vi "test - click2.vi"() -> ()   [LabVIEW 2020]
uses:
  <vilib>/Utility/miscctls.llb/LVPositionTypeDef.ctl
  ui-testing.lvlib
  User32.dll
panel:
  out "Position":T1
  in  "OK Button":bool
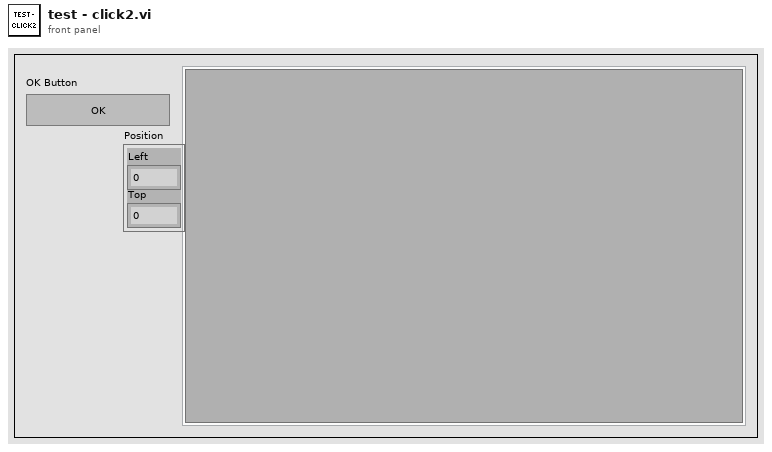
[diagram p1: front panel]
types:
  T1 = typedef "LVPositionTypeDef.ctl" = cluster{"Left":i32, "Top":i32}
  T2 = typedef "LVPointTypeDef.ctl" = cluster{"Horizontal":i16, "Vertical":i16}
  T3 = typedef "LVRectTypeDef.ctl" = cluster{"left":i16, "top":i16, "right":i16, "bottom":i16}
  T4 = typedef "LVBoundsTypeDef.ctl" = cluster{"Width":u32, "Height":u32}
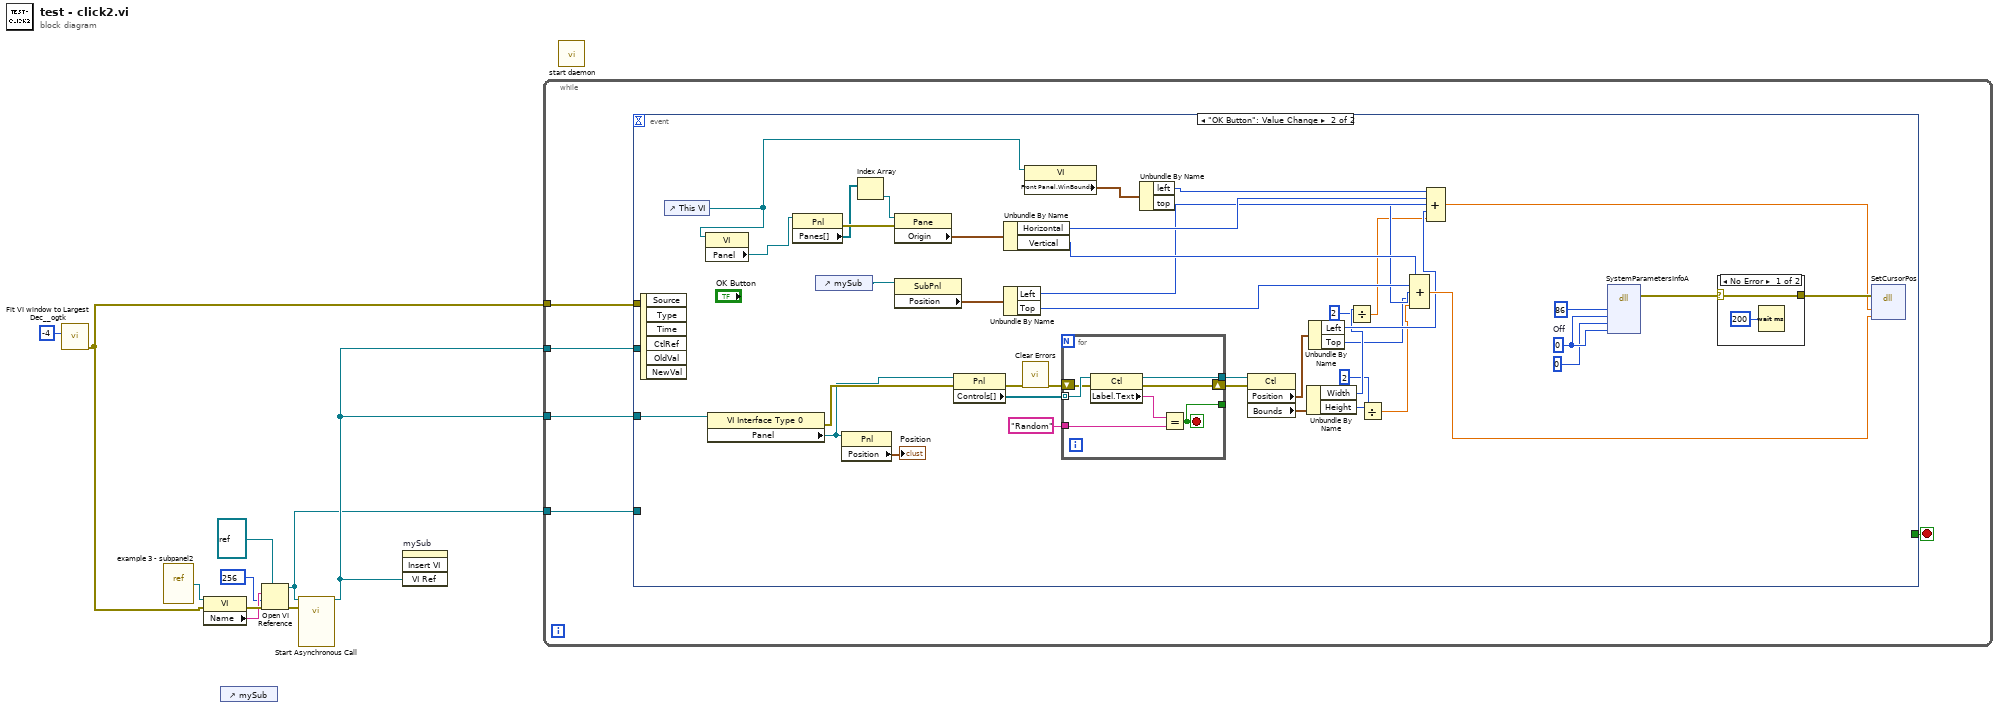
[diagram p0: block diagram]
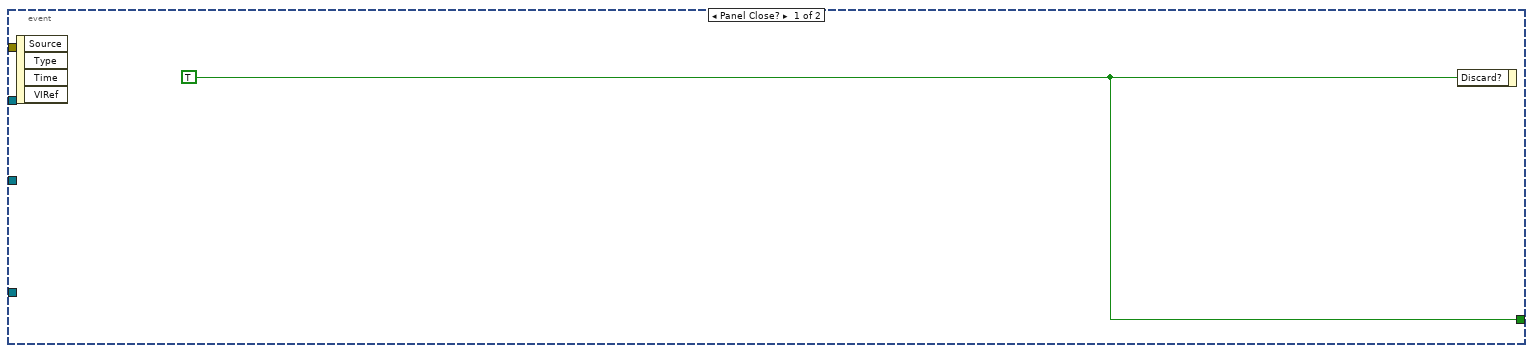
[diagram p2: hidden frame]
diagram:
  n1 = call <userlib>:"Fit VI window to Largest Dec__ogtk.vi"("border spacing (2 px)"=-4) -> ("error out"=w3:errorcluster)  [unwired: 5 in, 1 out]
  n2 = vi-ref "example 3 - subpanel2.vi"() -> (w8:refnum<vi>)
  n3 = property class="VI"(reference=w8, error in=w3) -> (error out=w10:errorcluster, "Name"=w9:string)  [unwired: 1 out]
  n4 = control-ref of="mySub"() -> ()  [unwired: 1 out]
  n5 = Open VI Reference(type specifier VI Refnum (for type only)=refnum<vi> refnum, vi path=w9, options=256 ("call and forget"), error in (no error)=w10) -> (vi reference=w1:refnum<vi>, error out=w7:errorcluster)  [unwired: 2 in]
  n6 = call-by-ref "Start Asynchronous Call"(reference=w1, error in=w7) -> (reference out=w2:refnum<vi>)  [unwired: 12 in, 1 out]
  n7 = invoke on="mySub" class="SubPnl" method="Insert VI"("VI Ref"=w2) -> ()  [unwired: 3 in, 4 out]
  n8 = while {
    tunnel: w3 -> [w14]
    tunnel: w2 -> [w13]
    tunnel: w2 -> [w12]
    tunnel: w1 -> [w11]
    stop <- w15 stop-if-true
    n9 = event shown="[1] \"OK Button\": Value Change" {
      selector: _ -> [_ _]
      dyn-events: _ -> [_ _]
      timeout: _ -> [_ _]
      tunnel: [w16 _] -> w15
      tunnel: w14 -> [_ _]
      tunnel: w13 -> [_ _]
      tunnel: w12 -> [_ w58]
      tunnel: w11 -> [_ _]
      event Panel Close? {
        w16 = TRUE
        n10 = event-data() -> ()  [unwired: 1 in, 4 out]
        n11 = event-data("Discard?"=w16) -> ()  [unwired: 1 in, 1 out]
      }
      event "OK Button": Value Change {
        w47 = u32 0  # Off
        n12 = event-data() -> ()  [unwired: 1 in, 6 out]
        n13 = control-ref of="This VI"() -> (w30:refnum<vi>)
        n14 = property class="VI"(reference=w30) -> ("Panel"=w39:refnum<vi>)  [unwired: 1 in, 2 out]
        n15 = property class="VI Interface Type 0"(reference=w58) -> (error out=w53:errorcluster, "Panel"=w49:refnum<vi>)  [unwired: 1 in, 1 out]
        n16 = property class="Pnl"(reference=w39) -> (error out=w42:errorcluster, "Panes[]"=w41:refnum<vi>[])  [unwired: 1 in, 1 out]
        n17 = control-ref of="mySub"() -> (w57:refnum<vi>)
        n18 = property class="Pnl"(reference=w49) -> ("Position"=→"Position":T1)  [unwired: 1 in, 2 out]
        n19 = Index Array(array=w41) -> (element=w40:refnum<vi>)  [unwired: 1 in]
        n20 = property class="Pane"(reference=w40, error in=w42) -> ("Origin"=w38:T2)  [unwired: 2 out]
        n21 = property class="SubPnl"(reference=w57) -> ("Position"=w37:T1)  [unwired: 1 in, 2 out]
        n22 = property class="Pnl"(reference=w49, error in=w53) -> (error out=w55:errorcluster, "Controls[]"=w56:refnum<vi>[])  [unwired: 1 out]
        n23 = Unbundle By Name(w38) -> ("Horizontal"=w36:i16, "Vertical"=w35:i16)
        n24 = Unbundle By Name(w37) -> ("Left"=w34:i32, "Top"=w33:i32)
        n25 = call <vilib>:"Clear Errors.vi"("error in (no error)"=w55) -> ("error out"=w54:errorcluster)  [unwired: 5 in, 1 out]
        n26 = property class="VI"(reference=w30) -> ("Front Panel.WinBounds"=w29:T3)  [unwired: 1 in, 2 out]
        n27 = for {
          tunnel: w56 -> [w68] mode=indexing
          tunnel: "Random" ("Control Label") -> [w66]
          tunnel: [w65] -> w51
          shift-right: [w63] -> w50
          shift-left: w54 -> [w64]
          tunnel: [w62] -> _
          stop <- w62 stop-if-true
          n28 = property class="Ctl"(reference=w68, error in=w64) -> (reference out=w65:refnum<vi>, error out=w63:errorcluster, "Label.Text"=w67:string)
          n29 = Equal?(x=w67, y=w66) -> (x = y?=w62:bool)
        }
        n30 = Unbundle By Name(w29) -> ("left"=w28:i16, "top"=w27:i16)
        n31 = property class="Ctl"(reference=w51, error in=w50) -> ("Position"=w26:T1, "Bounds"=w25:T4)  [unwired: 2 out]
        n32 = Unbundle By Name(w25) -> ("Width"=w23:u32, "Height"=w21:u32)
        n33 = Unbundle By Name(w26) -> ("Left"=w24:i32, "Top"=w22:i32)
        n34 = Divide(x=w23, y=u32 2) -> (x/y=w20:dbl)
        n35 = Divide(x=w21, y=u32 2) -> (x/y=w18:dbl)
        n36 = Compound Arithmetic op=ADD(w35, w33, w27, w22, w18) -> (w31:dbl)
        n37 = Compound Arithmetic op=ADD(w28, w36, w34, w24, w20) -> (w32:dbl)
        n38 = dll-call lib="User32.dll" fn="SystemParametersInfoA" label="Terminate power-off mode"("uiAction"=u32 86 ("SPI_GETPOWEROFFACTIVE"), "uiParam"=w47, "pvParam"=0, "fWinIni"=w47) -> (error out=w44:errorcluster)  [unwired: 8 in, 1 out]
        n39 = case shown="No Error" w44 {
          selector: w44 -> [w59 w61]
          tunnel: [w59 w61] -> w43
          frame No Error {
            n40 = Wait (ms)(milliseconds to wait=u32 200) -> ()  [unwired: 1 out]
          }
          frame Error {
          }
        }
        n41 = dll-call lib="User32.dll" fn="SetCursorPos" label="Move mouse"(error in=w43, "dx"=w32, "dy"=w31) -> ()  [unwired: 5 in, 2 out]
      }
    }
  }
  n42 = call "start daemon.vi"() -> ()  [unwired: 11 in, 1 out]
